vi "beginPassTo2ndStrikerPlay.vi"(8 "error in (no error)":errorcluster, 10 "Game":refnum<class "Game.lvclass">, 11 "PassTo2ndStriker in":refnum<class "PassTo2ndStriker.lvclass">) -> (0 "error out":errorcluster, 2 "beginPassTo2ndStriker?":bool, 3 "PassTo2ndStriker out":refnum<class "PassTo2ndStriker.lvclass">)   [LabVIEW 2020, in "PassTo2ndStriker.lvclass"]
uses:
  PassTo2ndStriker.lvclass
  Game_class/Game.lvclass
  Utilities_class/Utilities.lvclass
  Team_class/OffensivePlay.ctl
  Robot_class/roles.ctl
  Game_class/Game.lvclass/Game.ctl
  Referee_class/Referee.lvclass/Referee.ctl
  Referee_class/command_interpreted.ctl
  Team_class/Team.lvclass/Team.ctl
  Object_class/Object.lvclass/Object.ctl
  Object_class/Read x.vi
  Game_class/Read FieldRef.vi
  Game_class/Read Utilities.lvclass.vi
  Game_class/Read OffensiveTeam.vi
  Team_class/Read RobotRef.vi
  Team_class/Read OffensivePlay.vi
  Game_class/Read Referee.vi
  Referee_class/Read command_interpreted.vi
  Ally_class/Ally.lvclass
  C:/Users/anton/Desktop/RoboIME/IC/SSL_AI/Team_class/Team.lvclass
  Robot_class/Robot.lvclass
  C:/Users/anton/Desktop/RoboIME/IC/SSL_AI/Object_class/Object.lvclass
  Referee_class/Referee.lvclass
  Field_class/Field.lvclass
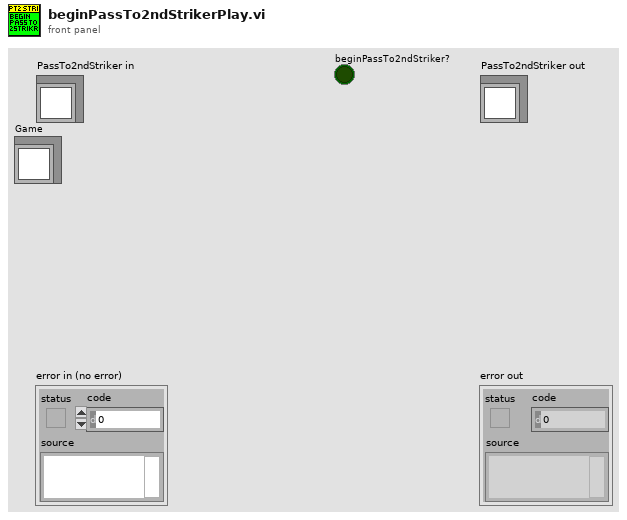
[diagram p1: front panel]
types:
  T1 = typedef "roles.ctl" = enum16{"SimpleBallPlacement", "BallPlacementAllyPasser", "BallPlacementAllyReceiver", "BallPlacementEnemy", "5Robots5th", "PassBestReceiver", "5Robots4th", "5Robots3rd", "5Robots2nd", "5Robots1st", "PassBestRobot", "WaitPass", "ABCThirdKicker", "ABCFirstKicker", "ABCSecondKicker", "Tabler", "TableFinalizer", "PrepareRollToPassRoller", "PrepareRollToPassReceiver", "SimplePassRoll", "SimplePassRollReceiver", "PenaltyDefense", "PreparePassReceiver 2", "PreparePassReceiver 1", "PassObserver", "Timeout", "Goto", "ZigZag", "None", "BallOutOfField", "DefenderArea", "Duelist", "AttackerStop", "FollowAttacker", "KeeperRole", "KickPenalty", "AttackerAimGoal", "AttackerBlock", "Marker", "Halt", "Shoot", "PassKicker", "PassReceiver", "TestRole", "PenaltyAttacker"}
  T2 = typedef "command_interpreted.ctl" = enum16{"Goal Ally", "Goal Enemy", "Ball Placement Enemy", "Ball Placement Ally", "Normal Half Time", "Extra Time  Break", "Extra Half Time", "None", "Post Game", "PKA Normal Start", "Prepare Kickoff Ally", "PKE Normal Start", "Prepare Kickoff Enemy", "Force Start", "Halt", "Timeout", "Prepare Penalty Ally", "Prepare Penalty Enemy", "PPA NormalStart", "PPE Normal Start", "Indirect Free Ally", "Direct Free Enemy", "Direct Free Ally", "Indirect Free Enemy", "Stop"}
  T3 = typedef "OffensivePlay.ctl" = enum16{"5RobotsPassGamePlay", "5PreparePassGame", "5RobotsKeeperGame", "KeeperPassToStriker", "5RobotsNormalGamePlay", "PrepareKeeperPass", "ACBPass", "ABCPass", "PrepareTriplePass", "TableWithStriker", "TableWith2ndStrikerPlay", "PrepareDoublePass", "PrepareRollToPass", "SimplePass", "PreparePass", "PassToStriker", "BallOutOfField", "PassTo2ndStriker", "StopOffensive", "Prepare Penalty Enemy", "EnemyPossessionAtEnemyField", "EnemyPossesionAtOurField", "TestPlay", "PreparePenaltyAlly", "KickPenaltyAlly", "PrepareKickoffAlly", "PrepareKickoffEnemy", "IndirectEnemy", "DirectEnemy", "PreparePassInGame1", "NormalGame", "DirectKick", "Pass", "Halt", "Timeout", "PassPlay", "PenaltyEnemy"}
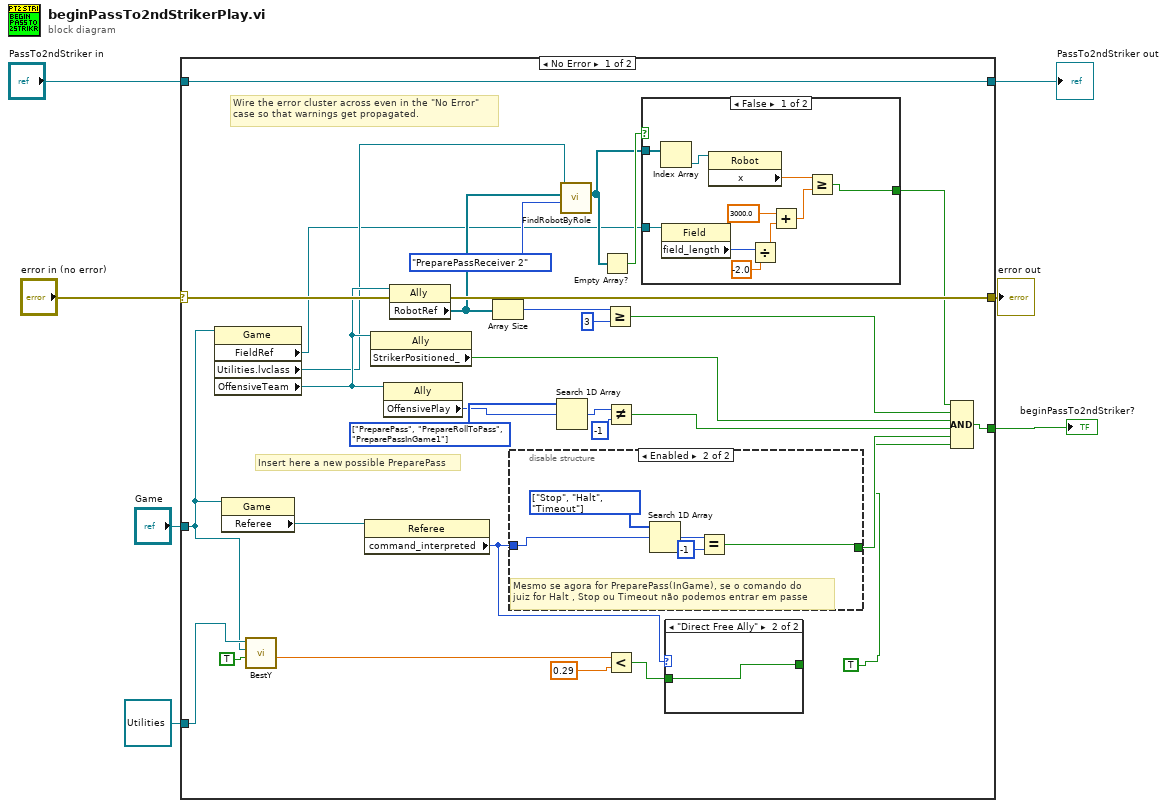
[diagram p0: block diagram]
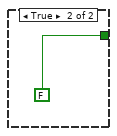
[diagram p2: hidden frame]
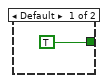
[diagram p3: hidden frame]
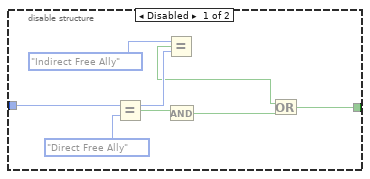
[diagram p4: hidden frame]
diagram:
  n1 = case shown="No Error" "error in (no error)" {
    selector: "error in (no error)" -> [w36 w64]
    tunnel: [w36 w64] -> w6
    tunnel: [w37 w63] -> w4
    tunnel: "PassTo2ndStriker in" -> [w37 w63]
    tunnel: "Game" -> [w16 _]
    tunnel: refnum<class "Utilities.lvclass"> refnum ("Utilities.lvclass") -> [w17 _]
    tunnel: [w19 _] -> w1
    frame No Error {
      w26 = T3[] [enum."PreparePass", enum."PrepareRollToPass", enum."PreparePassInGame1"] items=["5RobotsPassGamePlay", "5PreparePassGame", "5RobotsKeeperGame", "KeeperPassToStriker", "5RobotsNormalGamePlay", "PrepareKeeperPass", "ACBPass", "ABCPass", "PrepareTriplePass", "TableWithStriker", "TableWith2ndStrikerPlay", "PrepareDoublePass", "PrepareRollToPass", "SimplePass", "PreparePass", "PassToStriker", "BallOutOfField", "PassTo2ndStriker", "StopOffensive", "Prepare Penalty Enemy", "EnemyPossessionAtEnemyField", "EnemyPossesionAtOurField", "TestPlay", "PreparePenaltyAlly", "KickPenaltyAlly", "PrepareKickoffAlly", "PrepareKickoffEnemy", "IndirectEnemy", "DirectEnemy", "PreparePassInGame1", "NormalGame", "DirectKick", "Pass", "Halt", "Timeout", "PassPlay", "PenaltyEnemy"] ("Array")
      # "Insert here a new possible PreparePass"
      # "Wire the error cluster across even in the \"No Error\"\ncase so that warnings get propagated."
      n2 = property class="Game"(reference=w16) -> ("FieldRef"=w9:refnum<class "Field.lvclass">, "Utilities.lvclass"=w13:refnum<class "Utilities.lvclass">, "OffensiveTeam"=w18:refnum<class "Ally.lvclass">)  [unwired: 1 in, 2 out]
      n3 = property class="Game"(reference=w16) -> ("Referee"=w35:refnum<class "Referee.lvclass">)  [unwired: 1 in, 2 out]
      n4 = call "BestY.vi"("Utilities in"=w17, "Game"=w16, "inimigos"=TRUE) -> ("Gap kick"=w32:dbl)  [unwired: 2 in, 4 out]
      n5 = property class="Referee"(reference=w35) -> ("command_interpreted"=w21:T2)  [unwired: 1 in, 2 out]
      n6 = property class="Ally"(reference=w18) -> ("StrikerPositioned_"=w31:bool)  [unwired: 1 in, 2 out]
      n7 = property class="Ally"(reference=w18) -> ("OffensivePlay"=w25:T3)  [unwired: 1 in, 2 out]
      n8 = property class="Ally"(reference=w18) -> ("RobotRef"=w15:refnum<class "Robot.lvclass">[])  [unwired: 1 in, 2 out]
      n9 = Array Size(array=w15) -> (size(s)=w30:i32)
      n10 = disable-structure shown="Enabled" {
        disable-tunnel: w21 -> [w56 w62]
        disable-tunnel: [w51 w58] -> w27
        frame Disabled {
          n11 = Equal?(x=w56, y=command_interpreted."Direct Free Ally" ("command_interpreted")) -> (x = y?=w54:bool)
          n12 = Equal?(x=command_interpreted."Indirect Free Ally" ("command_interpreted"), y=w56) -> (x = y?=w52:bool)
          n13 = And(x=w54) -> (x .and. y?=w53:bool)  [unwired: 1 in]
          n14 = Or(x=w52, y=w53) -> (x .or. y?=w51:bool)
        }
        frame Enabled {
          w61 = T2[] [enum."Stop", enum."Halt", enum."Timeout"] items=["Goal Ally", "Goal Enemy", "Ball Placement Enemy", "Ball Placement Ally", "Normal Half Time", "Extra Time  Break", "Extra Half Time", "None", "Post Game", "PKA Normal Start", "Prepare Kickoff Ally", "PKE Normal Start", "Prepare Kickoff Enemy", "Force Start", "Halt", "Timeout", "Prepare Penalty Ally", "Prepare Penalty Enemy", "PPA NormalStart", "PPE Normal Start", "Indirect Free Ally", "Direct Free Enemy", "Direct Free Ally", "Indirect Free Enemy", "Stop"] ("1D array")
          # "Mesmo se agora for PreparePass(InGame), se o comando do\njuiz for Halt , Stop ou Timeout não podemos entrar em passe"
          n15 = Search 1D Array(1D array=w61, element=w62) -> (index of element=w60:i32)  [unwired: 1 in]
          n16 = Equal?(x=w60, y=-1) -> (x = y?=w58:bool)
        }
      }
      n17 = Search 1D Array(1D array=w26, element=w25) -> (index of element=w24:i32)  [unwired: 1 in]
      n18 = call "FindRobotByRole.vi"("role"=roles."PreparePassReceiver 2", "RobotRef"=w15, "Utilities in"=w13) -> ("Robots"=w10:refnum<class "Robot.lvclass">[])  [unwired: 6 in, 2 out]
      n19 = Empty Array?(array=w10) -> (empty?=w12:bool)
      n20 = Greater Or Equal?(x=w30, y=3) -> (x >= y?=w28:bool)
      n21 = Not Equal?(x=w24, y=-1) -> (x != y?=w22:bool)
      n22 = Less?(x=w32, y=0.29 ("Gap kick")) -> (x < y?=w20:bool)
      n23 = case shown="False" w12 {
        tunnel: [w44 FALSE] -> w11
        tunnel: w10 -> [w47 _]
        tunnel: w9 -> [w43 _]
        frame False {
          n24 = Index Array(array=w47) -> (element=w46:refnum<class "Robot.lvclass">)  [unwired: 1 in]
          n25 = property class="Field"(reference=w43) -> ("field_length"=w42:i32)  [unwired: 1 in, 2 out]
          n26 = property class="Robot"(reference=w46) -> ("x"=w45:dbl)  [unwired: 1 in, 2 out]
          n27 = Divide(x=w42, y=-2.0) -> (x/y=w40:dbl)
          n28 = Add(x=3000.0, y=w40) -> (x+y=w39:dbl)
          n29 = Greater Or Equal?(x=w45, y=w39) -> (x >= y?=w44:bool)
        }
        frame True {
        }
      }
      n30 = case shown="\"Direct Free Ally\"" w21 {
        tunnel: [TRUE w50] -> _
        tunnel: w20 -> [_ w50]
        frame Default {
        }
        frame "Direct Free Ally" {
        }
      }
      n31 = Compound Arithmetic op=AND(w11, w28, w31, w22, w27, TRUE ("value")) -> (w19:bool)
    }
    frame Error {
    }
  }
  "error out" <- w6
  "PassTo2ndStriker out" <- w4
  "beginPassTo2ndStriker?" <- w1
